vi "Set and Get Manipulator Position.vi"(8 "error in (no error)":errorcluster, 10 "Numeric in":dbl, 11 "Primary Scan Manipulator Axis":i32) -> (0 "error out":errorcluster, 3 "Numeric out":dbl)   [LabVIEW 2020, in "Acquisition Example.lvlib"]
uses:
  Acquisition Example.lvlib
  Manipulator-DQMH/Libraries/Manipulator/Manipulator.lvlib
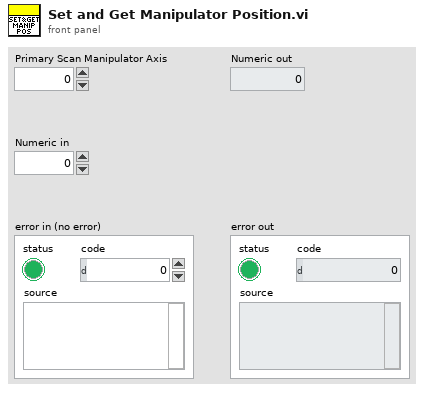
[diagram p1: front panel]
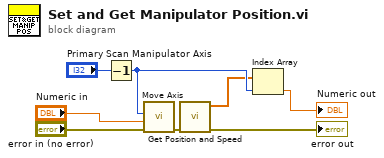
[diagram p0: block diagram]
diagram:
  n1 = Decrement(x="Primary Scan Manipulator Axis") -> (x-1=w7:i32)
  n2 = call "Move Axis.vi"("error in"="error in (no error)", "Position"="Numeric in", "Axis"=w7) -> ("error out"=w2:errorcluster)  [unwired: 7 in, 1 out]
  n3 = call "Get Position and Speed.vi"("error in"=w2) -> ("error out"=→"error out":errorcluster, "Positions"=w6:dbl[])  [unwired: 7 in, 2 out]
  n4 = Index Array(array=w6, index=w7) -> (element=→"Numeric out":dbl)
